vi "BuildFarm INI Tool.vi"(7 "WorkerShow":bool=TRUE, 8 "error in (no error)":errorcluster, 9 "CommPort":u32=4545, 10 "WorkerFolder":path=path "/Volumes/Data/Users/benji667/Git/BuildFarm/src/BuildWorker", 11 "WorkerInterface":string="BuildWorker Basics.lvclass") -> (0 "error out":errorcluster, 3 "file path":path)   [LabVIEW 2017]
uses:
  <vilib>/Utility/config.llb/Write Key (U32).vi
  <vilib>/Utility/config.llb/Write Key (Boolean).vi
  <vilib>/Utility/config.llb/Write Key (Path).vi
  <vilib>/Utility/config.llb/Write Key (String).vi
  <vilib>/Utility/config.llb/NI_LVConfig.lvlib
panel:
  in  "ServerFolder":path=path "/Volumes/Data/Users/benji667/Git/BuildFarm/src/BuildServer"
  in  "ServerLauncher":string="BuildServer Launcher.vi"
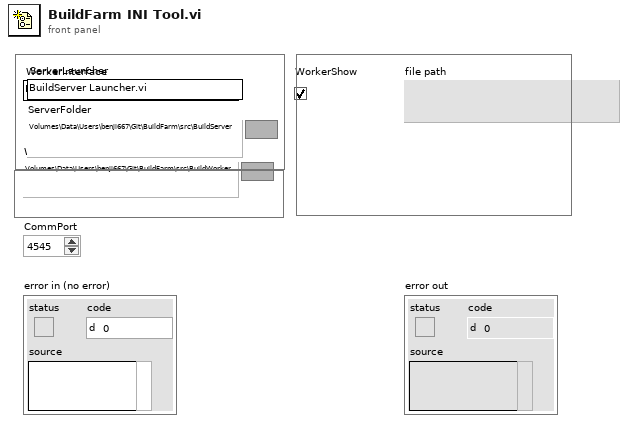
[diagram p1: front panel]
types:
  T1 = typedef "NI_LVConfig.lvlib/Config Data RefNum.ctl" = refnum<k1>
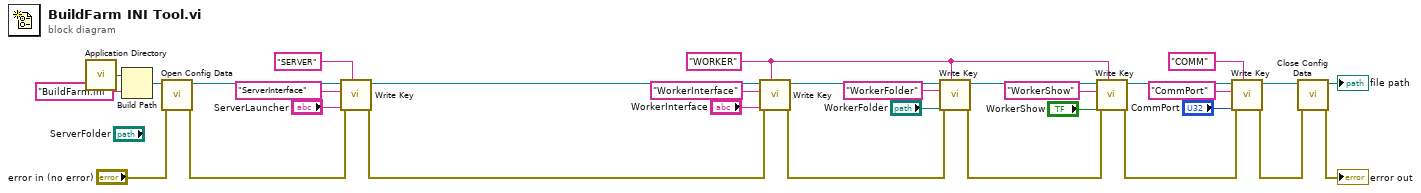
[diagram p0: block diagram]
diagram:
  w14 = "WORKER" ("section")
  n1 = call <vilib>:"Application Directory.vi"() -> ("Application Directory"=w31:path)
  n2 = Build Path(base path=w31, name or relative path="BuildFarm.ini") -> (appended path=w13:path)
  n3 = call <vilib>:"Open Config Data.vi"("error in (no error)"="error in (no error)", "configuration file path"=w13) -> ("error out"=w2:errorcluster, "refnum"=w4:T1)  [unwired: 7 in, 1 out]
  n4 = call-poly <vilib>:"Write Key.vi"("section"="SERVER", "error in (no error)"=w2, "value"="ServerLauncher", "key"="ServerInterface", "refnum"=w4) -> ("error out"=w1:errorcluster, "refnum out"=w3:T1)  [unwired: 4 in, 1 out]
  n5 = call-poly <vilib>:"Write Key.vi"("section"=w14, "error in (no error)"=w1, "value"="WorkerInterface", "key"="WorkerInterface", "refnum"=w3) -> ("error out"=w16:errorcluster, "refnum out"=w19:T1)  [unwired: 4 in, 1 out]
  n6 = call-poly <vilib>:"Write Key.vi"("section"=w14, "error in (no error)"=w16, "value"="WorkerFolder", "key"="WorkerFolder", "refnum"=w19) -> ("error out"=w15:errorcluster, "refnum out"=w18:T1)  [unwired: 4 in, 1 out]
  n7 = call-poly <vilib>:"Write Key.vi"("section"=w14, "error in (no error)"=w15, "value"="WorkerShow", "key"="WorkerShow", "refnum"=w18) -> ("error out"=w24:errorcluster, "refnum out"=w25:T1)  [unwired: 4 in, 1 out]
  n8 = call-poly <vilib>:"Write Key.vi"("section"="COMM", "error in (no error)"=w24, "value"="CommPort", "key"="CommPort", "refnum"=w25) -> ("error out"=w22:errorcluster, "refnum out"=w23:T1)  [unwired: 4 in, 1 out]
  n9 = call <vilib>:"Close Config Data.vi"("error in (no error)"=w22, "refnum"=w23) -> ("error out"=→"error out":errorcluster, "file path"=→"file path":path)  [unwired: 8 in]
